vi "TS DAC Run Stop.vi"(8 "error in (no error)":errorcluster, 11 "Heat Flow Test Stand in":refnum<class "Heat Flow Test Stand.lvclass">) -> (0 "error out":errorcluster, 3 "Heat Flow Test Stand out":refnum<class "Heat Flow Test Stand.lvclass">)   [LabVIEW 2019, in "Test Stands.lvlib" / "Heat Flow Test Stand.lvclass"]
uses:
  Heat Flow Test Stand.lvclass
  Generic Test Stand/Generic Test Stand.lvclass
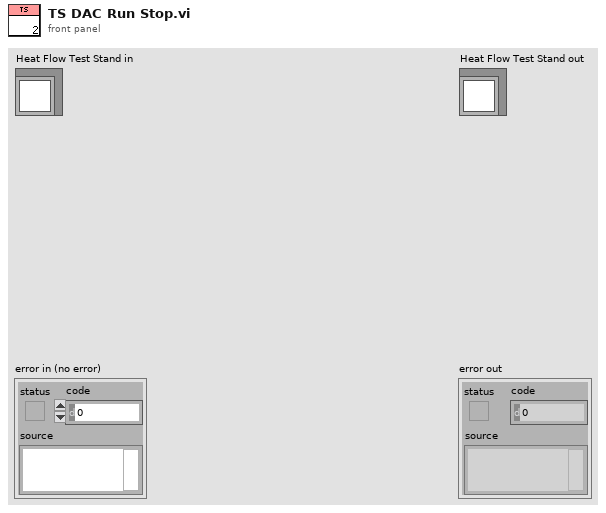
[diagram p1: front panel]
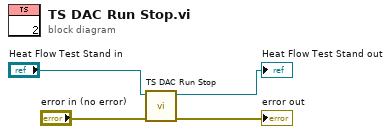
[diagram p0: block diagram]
diagram:
  n1 = call-parent "TS DAC Run Stop.vi"("error in (no error)"="error in (no error)", "Generic Test Stand in"="Heat Flow Test Stand in") -> ("error out"=→"error out":errorcluster, "Generic Test Stand out"=→"Heat Flow Test Stand out":refnum<class "Heat Flow Test Stand.lvclass">)  [unwired: 8 in]
